vi "Range_To_Mult.vi"(10 "Range":T1(ring)) -> (1 "Unit":string, 2 "Mult":dbl)   [LabVIEW 2013]
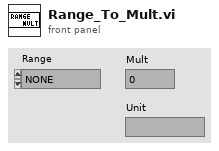
[diagram p1: front panel]
types:
  T1 = enum16{"NONE", "1MV", "2MV", "5MV", "10MV", "20MV", "50MV", "100MV", "200MV", "500MV", "1V", "2V", "5V", "10V", "20V", "50V", "100V", "200V", "500V", "1KV", "1-5V", "TCK", "TCJ", "TCT", "TCR", "TCE", "TCB", "TCS", "TCN", "TCW", "PT100", "JPT100", "PT1000", "400UE", "500UE", "800UE", "1000UE", "2000UE", "4000UE", "5000UE", "8000UE", "10000UE", "20000UE", "0.2MVPV", "0.25MVPV", "0.4MVPV", "0.5MVPV", "1MVPV", "2MVPV", "2.5MVPV", "4MVPV", "5MVPV", "10MVPV", "1OHM", "2OHM", "5OHM", "10OHM", "20OHM", "50OHM", "100OHM", "200OHM", "500OHM", "1KOHM", "2KOHM", "5KOHM", "10KOHM", "20KOHM", "50KOHM", "1MPSS", "2MPSS", "5MPSS", "10MPSS", "20MPSS", "50MPSS", "100MPSS", "200MPSS", "500MPSS", "1000MPSS", "2000MPSS", "5000MPSS", "10000MPSS", "20000MPSS", "50000MPSS", "200MPA", "400MPA", "500MPA", "1PA", "2PA", "4PA", "5PA", "10PA", "20PA", "40PA", "50PA", "100PA", "200PA", "400PA", "500PA"}
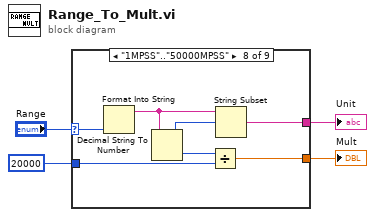
[diagram p0: block diagram]
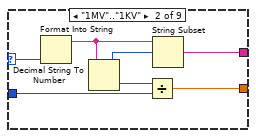
[diagram p3: hidden frame]
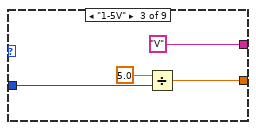
[diagram p4: hidden frame]
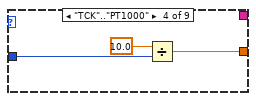
[diagram p5: hidden frame]
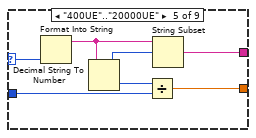
[diagram p6: hidden frame]
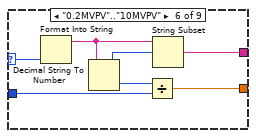
[diagram p7: hidden frame]
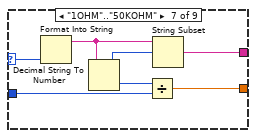
[diagram p8: hidden frame]
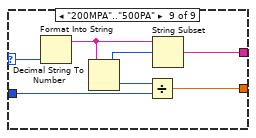
[diagram p9: hidden frame]
diagram:
  n1 = case shown="\"1MPSS\"..\"50000MPSS\"" "Range" {
    selector: "Range" -> [_ w11 _ _ w25 w32 w39 w46 w53]
    tunnel: 20000 -> [_ w9 w14 w17 w23 w30 w37 w44 w51]
    tunnel: [_ w8 w13 w16 w22 w29 w36 w43 w50] -> w2
    tunnel: [_ w5 "V" _ w20 w26 w34 w41 w49] -> w1
    frame "NONE" {
    }
    frame "1MV".."1KV" {
      n2 = Format Into String(w11) -> (resulting string=w7:string)  [unwired: 3 in, 1 out]
      n3 = Decimal String To Number(string=w7) -> (offset past number=w6:i32, number=w10:i32)  [unwired: 2 out]
      n4 = Divide(x=w10, y=w9) -> (x/y=w8:dbl)
      n5 = String Subset(string=w7, offset (0)=w6) -> (substring=w5:string)  [unwired: 1 in]
    }
    frame "1-5V" {
      n6 = Divide(x=5.0, y=w14) -> (x/y=w13:dbl)
    }
    frame "TCK".."PT1000" {
      n7 = Divide(x=10.0, y=w17) -> (x/y=w16:dbl)
    }
    frame "400UE".."20000UE" {
      n8 = Format Into String(w25) -> (resulting string=w21:string)  [unwired: 3 in, 1 out]
      n9 = Decimal String To Number(string=w21) -> (offset past number=w19:i32, number=w24:i32)  [unwired: 2 out]
      n10 = Divide(x=w24, y=w23) -> (x/y=w22:dbl)
      n11 = String Subset(string=w21, offset (0)=w19) -> (substring=w20:string)  [unwired: 1 in]
    }
    frame "0.2MVPV".."10MVPV" {
      n12 = Format Into String(w32) -> (resulting string=w27:string)  [unwired: 3 in, 1 out]
      n13 = Decimal String To Number(string=w27) -> (offset past number=w28:i32, number=w31:i32)  [unwired: 2 out]
      n14 = Divide(x=w31, y=w30) -> (x/y=w29:dbl)
      n15 = String Subset(string=w27, offset (0)=w28) -> (substring=w26:string)  [unwired: 1 in]
    }
    frame "1OHM".."50KOHM" {
      n16 = Format Into String(w39) -> (resulting string=w35:string)  [unwired: 3 in, 1 out]
      n17 = Decimal String To Number(string=w35) -> (offset past number=w33:i32, number=w38:i32)  [unwired: 2 out]
      n18 = Divide(x=w38, y=w37) -> (x/y=w36:dbl)
      n19 = String Subset(string=w35, offset (0)=w33) -> (substring=w34:string)  [unwired: 1 in]
    }
    frame "1MPSS".."50000MPSS" {
      n20 = Format Into String(w46) -> (resulting string=w42:string)  [unwired: 3 in, 1 out]
      n21 = Decimal String To Number(string=w42) -> (offset past number=w40:i32, number=w45:i32)  [unwired: 2 out]
      n22 = Divide(x=w45, y=w44) -> (x/y=w43:dbl)
      n23 = String Subset(string=w42, offset (0)=w40) -> (substring=w41:string)  [unwired: 1 in]
    }
    frame "200MPA".."500PA" {
      n24 = Format Into String(w53) -> (resulting string=w48:string)  [unwired: 3 in, 1 out]
      n25 = Decimal String To Number(string=w48) -> (offset past number=w47:i32, number=w52:i32)  [unwired: 2 out]
      n26 = Divide(x=w52, y=w51) -> (x/y=w50:dbl)
      n27 = String Subset(string=w48, offset (0)=w47) -> (substring=w49:string)  [unwired: 1 in]
    }
  }
  "Mult" <- w2
  "Unit" <- w1
